vi "MotorAxisNotifier.vi"(1 "Status":enum16{"OFF", "IDLE", "MOVING", "HOMING"}(ring), 2 "New Motor Name":string, 3 "COM Port in":refnum<visa-resource-name>, 4 "Previous Motor Name":string, 5 "MotorData":T1[](array[typedef]), 7 "Update Position?":bool, 8 "occurrence":refnum<k4>, 9 "error in (no error)":errorcluster) -> (0 "COM Port out":refnum<visa-resource-name>, 6 "error out":errorcluster)   [LabVIEW 2009]
uses:
  Controls/MotorData.ctl
  Controls/MotorNamedPosition.ctl
  Controls/MotorStatus.ctl
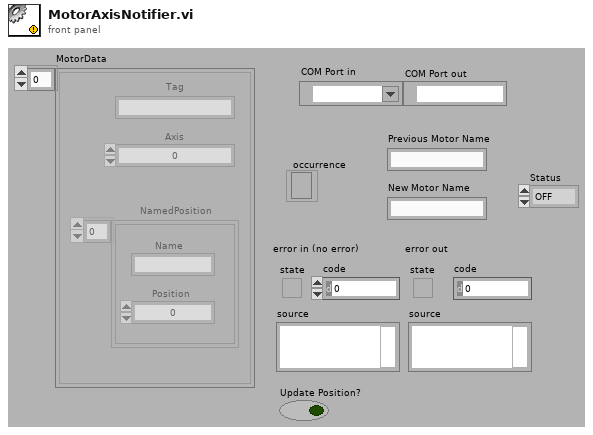
[diagram p1: front panel]
types:
  T1 = typedef "MotorData.ctl" = cluster{"Tag":string, "Axis":i32, "NamedPosition":T2[]}
  T2 = typedef "MotorNamedPosition.ctl" = cluster{"Position":i32, "Name":string}
  T3 = typedef "MotorStatus.ctl" = cluster{"Managed?":bool, "Position":i32, "Name":string, "Status":enum16{"OFF", "IDLE", "MOVING", "HOMING"}}
  T4 = enum16{"?SEL", "?POS", "?VMIN", "?VMAX", "?ACC", "?MPAS", "?INT", "?JEU", "?OFFSET", "?L", "?FDC", "??", "?ST", "?MVT"}
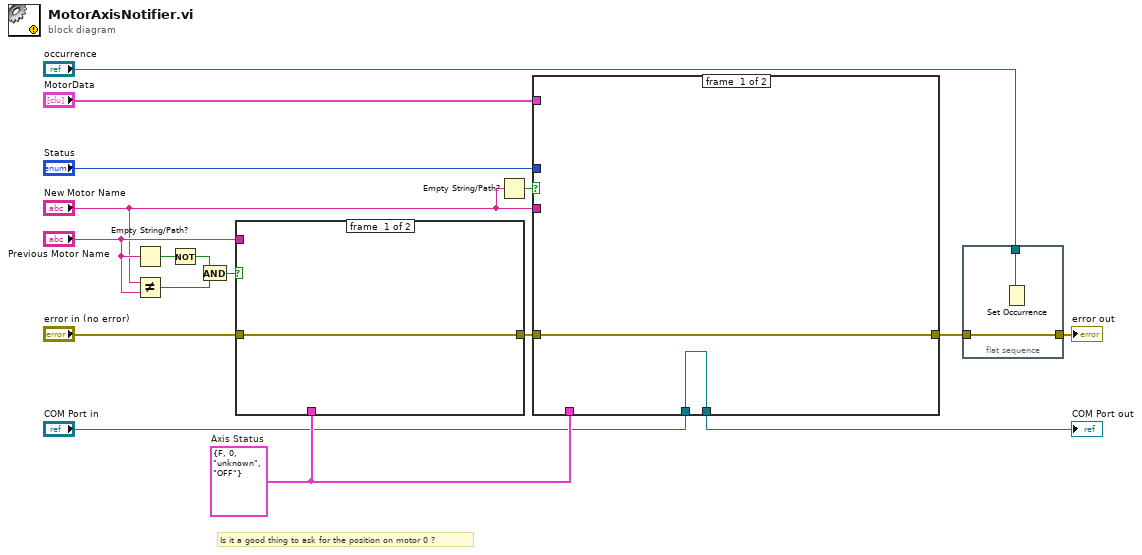
[diagram p0: block diagram]
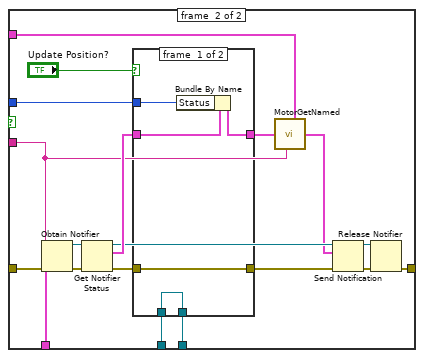
[diagram p2: hidden frame]
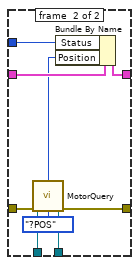
[diagram p3: hidden frame]
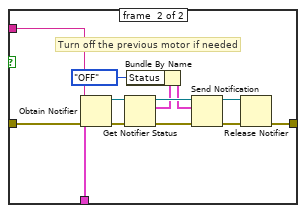
[diagram p4: hidden frame]
diagram:
  w16 = T3 {"Managed?"=FALSE, "Position"=0, "Name"="unknown", "Status"=enum."OFF"}  # Axis Status
  # "Is it a good thing to ask for the position on motor 0 ?"
  n1 = Empty String/Path?(string/path="Previous Motor Name") -> (empty?=w14:bool)
  n2 = Not Equal?(x="New Motor Name", y="Previous Motor Name") -> (x != y?=w13:bool)
  n3 = Not(x=w14) -> (.not. x?=w10:bool)
  n4 = And(x=w10, y=w13) -> (x .and. y?=w12:bool)
  n5 = case shown="True" w12 {
    tunnel: "error in (no error)" -> [w18 w20]
    tunnel: w16 -> [_ w25]
    tunnel: "Previous Motor Name" -> [_ w21]
    tunnel: [w18 w22] -> w17
    frame #0 {
    }
    frame #1 {
      # "Turn off the previous motor if needed"
      n6 = Obtain Notifier(name (unnamed)=w21, notification data type=w25, error in (no error)=w20) -> (notifier out=w31:refnum<notifier>, error out=w19:errorcluster)  [unwired: 1 in, 1 out]
      n7 = Get Notifier Status(notifier=w31, error in (no error)=w19) -> (notifier out=w30:refnum<notifier>, current notification=w28:T3, error out=w29:errorcluster)  [unwired: 2 out]
      n8 = Bundle By Name(cluster=w28, "Status"=enum16{"OFF", "IDLE", "MOVING", "HOMING"}."OFF") -> (w27:T3)
      n9 = Send Notification(notification=w27, notifier=w30, error in (no error)=w29) -> (notifier out=w23:refnum<notifier>, error out=w24:errorcluster)
      n10 = Release Notifier(notifier=w23, error in (no error)=w24) -> (error out=w22:errorcluster)  [unwired: 3 out]
    }
  }
  n11 = Empty String/Path?(string/path="New Motor Name") -> (empty?=w1:bool)
  n12 = case shown="False" w1 {
    tunnel: w17 -> [w33 w44]
    tunnel: w16 -> [_ w49]
    tunnel: [w33 w45] -> w9
    tunnel: "Status" -> [_ w48]
    tunnel: "COM Port in" -> [w32 w43]
    tunnel: [w32 w42] -> w4
    tunnel: "MotorData" -> [_ w36]
    tunnel: "New Motor Name" -> [_ w35]
    frame #0 {
    }
    frame #1 {
      n13 = Obtain Notifier(name (unnamed)=w35, notification data type=w49, error in (no error)=w44) -> (notifier out=w50:refnum<notifier>, error out=w34:errorcluster)  [unwired: 1 in, 1 out]
      n14 = Get Notifier Status(notifier=w50, error in (no error)=w34) -> (notifier out=w51:refnum<notifier>, current notification=w52:T3, error out=w40:errorcluster)  [unwired: 2 out]
      n15 = case shown="False" "Update Position?" {
        tunnel: [w54 w66] -> w38
        tunnel: w52 -> [w55 w65]
        tunnel: w48 -> [w53 w64]
        tunnel: w43 -> [w57 w61]
        tunnel: [w57 w60] -> w42
        tunnel: w40 -> [w56 w59]
        tunnel: [w56 w58] -> w39
        frame #0 {
          n16 = Bundle By Name(cluster=w55, "Status"=w53) -> (w54:T3)
        }
        frame #1 {
          n17 = call "MotorQuery.vi"("VISA in"=w61, "Command"=T4."?POS", "entrée d'erreur"=w59) -> ("VISA out"=w60:refnum<visa-resource-name>, "I32 Result"=w62:i32, "sortie d'erreur"=w58:errorcluster)  [unwired: 4 out]
          n18 = Bundle By Name(cluster=w65, "Status"=w64, "Position"=w62) -> (w66:T3)
        }
      }
      n19 = call "MotorGetNamed.vi"("Motor status in"=w38, "MotorName"=w35, "MotorData"=w36) -> ("Motor status out"=w37:T3)
      n20 = Send Notification(notification=w37, notifier=w51, error in (no error)=w39) -> (notifier out=w47:refnum<notifier>, error out=w46:errorcluster)
      n21 = Release Notifier(notifier=w47, error in (no error)=w46) -> (error out=w45:errorcluster)  [unwired: 3 out]
    }
  }
  "COM Port out" <- w4
  n22 = flat-sequence {
    tunnel: w9 -> [w68]
    tunnel: [w68] -> w8
    tunnel: "occurrence" -> [w67]
    frame #0 {
      n23 = Set Occurrence(w67) -> ()
    }
  }
  "error out" <- w8
